vi "Get All Controls Value And Type.vi"(8 "错误输入（无错误）":errorcluster, 10 "Select":enum16{"Control", "Indicator"}(ring), 11 "VI Ref":refnum<vi>) -> (0 "错误输出":errorcluster, 2 "Enum Types":T1[](array[typedef]), 3 "All Control Value":cluster{"Name":string, "Variant Data":variant}[](array[cluster]))   [LabVIEW 2012, in "VIRef.lvlib"]
uses:
  VIRef.lvlib
  <vilib>/Utility/VariantDataType/Type.ctl
  <vilib>/Utility/VariantDataType/VariantType.lvlib
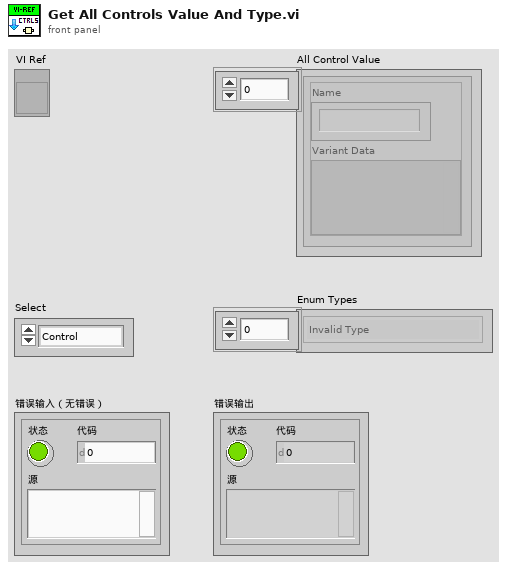
[diagram p1: front panel]
types:
  T1 = typedef "VariantType.lvlib/Type.ctl" = enum8{"Invalid Type", "Void", "I8", "I16", "I32", "I64", "U8", "U16", "U32", "U64", "Single Float", "Double Float", "Extended Float", "Single Complex", "Double Complex", "Extended Complex", "Enum U8", "Enum U16", "Enum U32", "Enum U64", "Single Float With Unit", "Double Float With Unit", "Extended Float With Unit", "Single Complex with Unit", "Double Complex with Unit", "Extended Complex with Unit", "Boolean", "String", "Path", "Picture", "Tag", "Array", "Cluster", "Variant", "LV Variant", "Waveform", "Timestamp", "Digital Waveform", "Digital Data", "ExpressData", "Refnum", "External Data", "VI", "Poly VI", "LabVIEW Class Instance", "Fixed Point"}
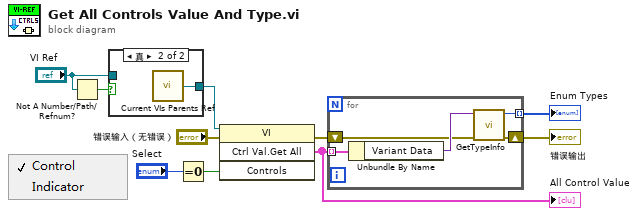
[diagram p0: block diagram]
diagram:
  n1 = Not A Number/Path/Refnum?(number/path/refnum="VI Ref") -> (NaN/Path/Refnum?=w9:bool)
  n2 = case shown="真" w9 {
    tunnel: [w11 w12] -> w8
    tunnel: "VI Ref" -> [w11 _]
    frame False {
    }
    frame True {
      n3 = call "Current VIs Parents Ref.vi"() -> ("Calling VI's Reference"=w12:refnum<vi>)  [unwired: 2 in]
    }
  }
  n4 = Equal To 0?(x="Select") -> (x = 0?=w6:bool)
  n5 = invoke class="VI" method="Ctrl Val.Get All"(reference=w8, error in="错误输入（无错误）", "Controls"=w6) -> (error out=w3:errorcluster, "Get All Control Values Variant"=w4:cluster{"Name":string, "Variant Data":variant}[])  [unwired: 1 in, 2 out]
  "All Control Value" <- w4
  n6 = for {
    tunnel: w4 -> [w17] mode=indexing
    shift-right: [w15] -> w1
    shift-left: w3 -> [w13]
    tunnel: [w14] -> w2 mode=indexing
    n7 = Unbundle By Name(w17) -> ("Variant Data"=w16:variant)
    n8 = call <vilib>:"GetTypeInfo.vi"("error in (no error)"=w13, "Variant"=w16) -> ("error out"=w15:errorcluster, "Type Enum"=w14:T1)  [unwired: 5 in, 3 out]
  }
  "错误输出" <- w1
  "Enum Types" <- w2
